vi "Check Transform-CV Status.vi"(8 "error in (no error)":errorcluster, 11 "transformCvToolkit in":refnum<class "transformCvToolkit.lvclass">) -> (0 "error out":errorcluster, 2 "status":string, 3 "transformCvToolkit out":refnum<class "transformCvToolkit.lvclass">)   [LabVIEW 2024, in "transformCvToolkit.lvclass"]
uses:
  transformCvToolkit.lvclass
  transformCvToolkit.lvclass/transformCvToolkit.ctl
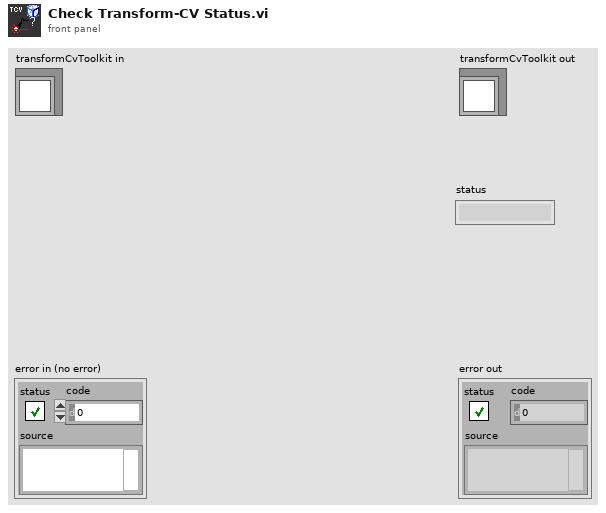
[diagram p1: front panel]
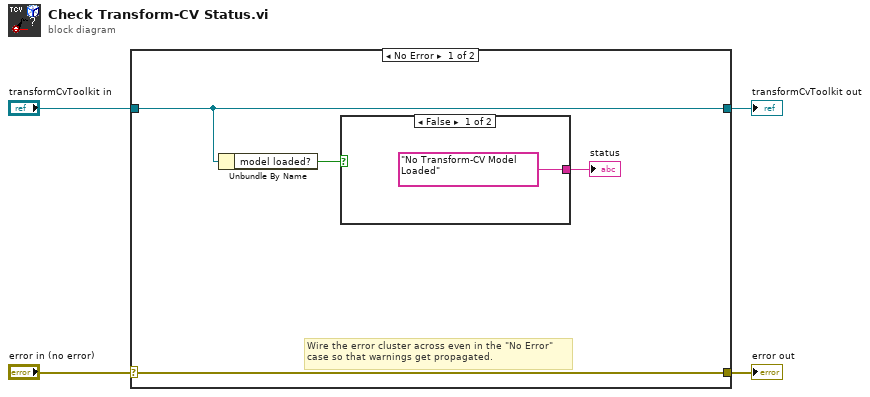
[diagram p0: block diagram]
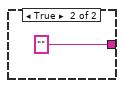
[diagram p2: hidden frame]
diagram:
  n1 = case shown="No Error" "error in (no error)" {
    selector: "error in (no error)" -> [w8 w12]
    tunnel: [w8 w12] -> w3
    tunnel: [w7 w11] -> w1
    tunnel: "transformCvToolkit in" -> [w7 w11]
    frame No Error {
      # "Wire the error cluster across even in the \"No Error\"\ncase so that warnings get propagated."
      n2 = Unbundle By Name(w7) -> ("model loaded?"=w6:bool)
      n3 = case shown="False" w6 {
        tunnel: ["No Transform-CV Model Loaded" ("status") "" ("status")] -> w5
        frame False {
        }
        frame True {
        }
      }
      "status" <- w5
    }
    frame Error {
    }
  }
  "error out" <- w3
  "transformCvToolkit out" <- w1
